vi "Program status info.vi"(8 "error in (no error)":errorcluster, 11 "ARS-0220 in":refnum<class "ARS-0220.lvclass">) -> (0 "error out":errorcluster, 3 "ARS-0220 out":refnum<class "ARS-0220.lvclass">)   [LabVIEW 2021, in "Environment Chamber.lvlib" / "ARS-0220.lvclass"]
uses:
  ARS-0220.lvclass
  Abstract/Abstract.lvclass
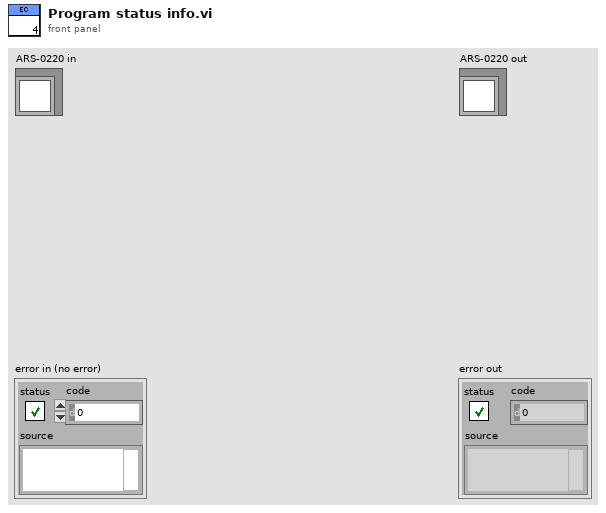
[diagram p1: front panel]
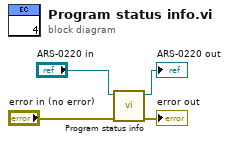
[diagram p0: block diagram]
diagram:
  n1 = call-parent "Program status info.vi"("error in (no error)"="error in (no error)", "Abstract in"="ARS-0220 in") -> ("error out"=→"error out":errorcluster, "Abstract out"=→"ARS-0220 out":refnum<class "ARS-0220.lvclass">)  [unwired: 8 in]
